vi "avgvi.vi"(11 "image in":sgl[][](array[numeric])) -> (3 "image out":sgl[][](array[numeric]))   [LabVIEW 2017]
doc: "SciScan 1.2 160622"
uses:
  GFG/GFGnumericGet.vi
  GFG/GFG library.lvlib
panel:
  in  "avg":sgl[][][](array[numeric])
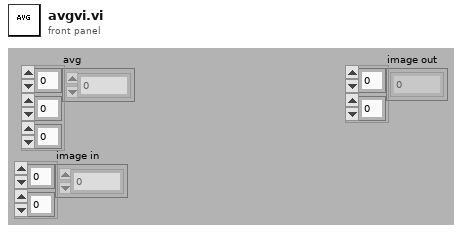
[diagram p1: front panel]
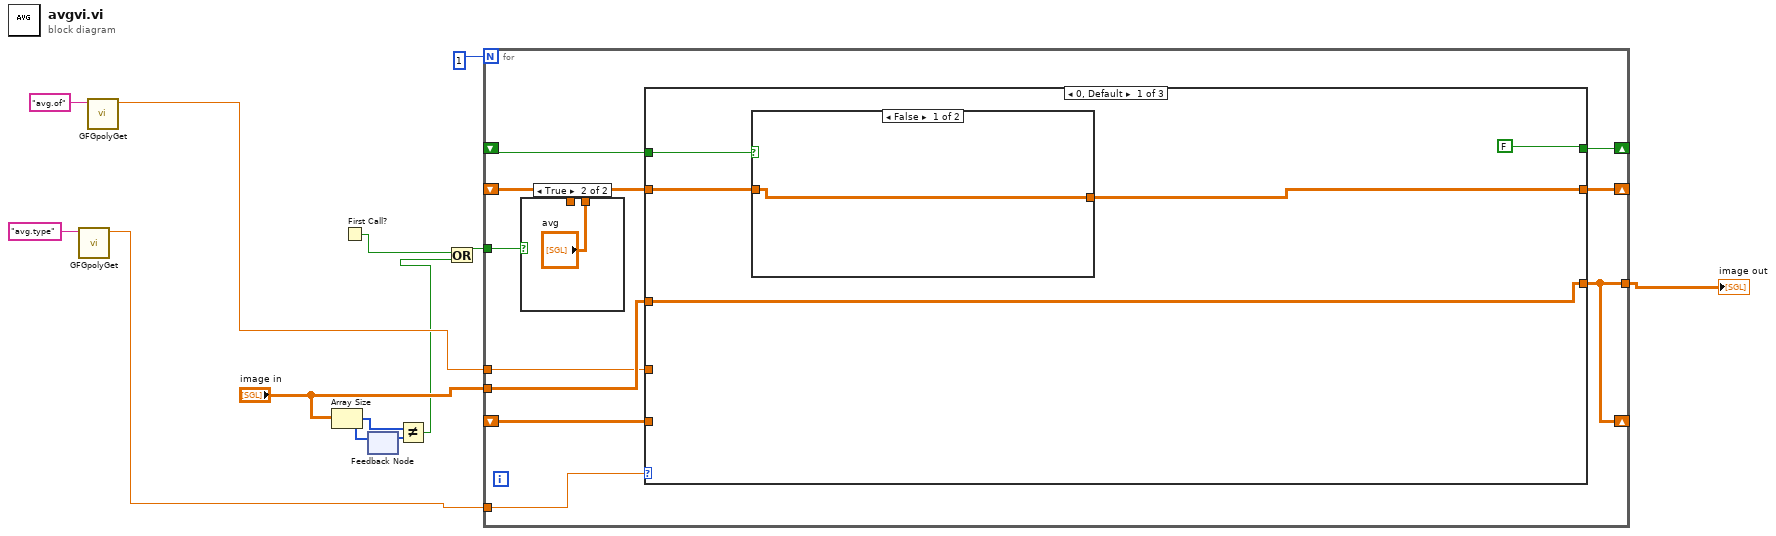
[diagram p0: block diagram]
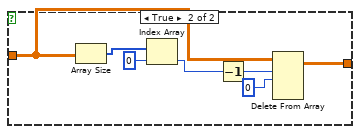
[diagram p2: hidden frame]
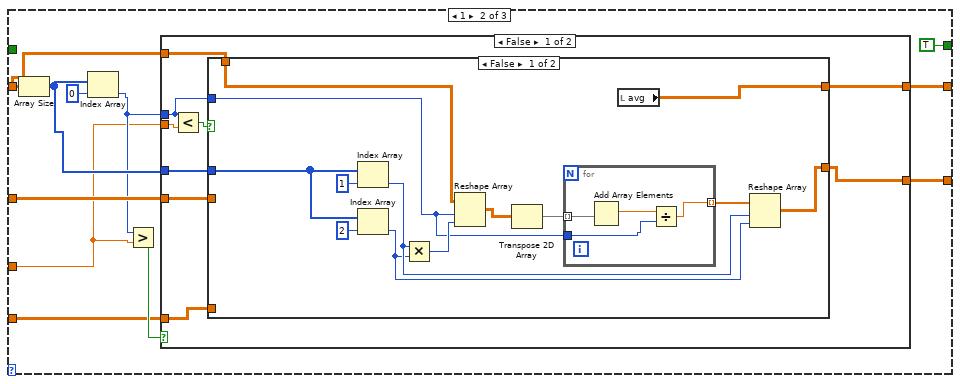
[diagram p3: hidden frame]
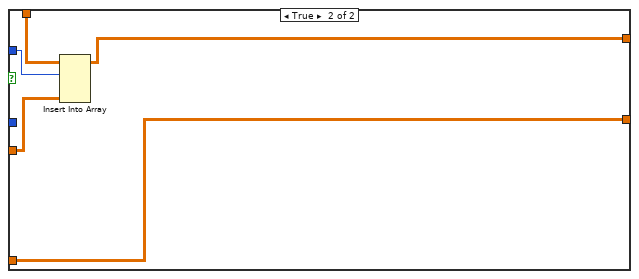
[diagram p4: hidden frame]
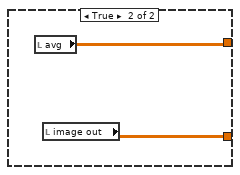
[diagram p5: hidden frame]
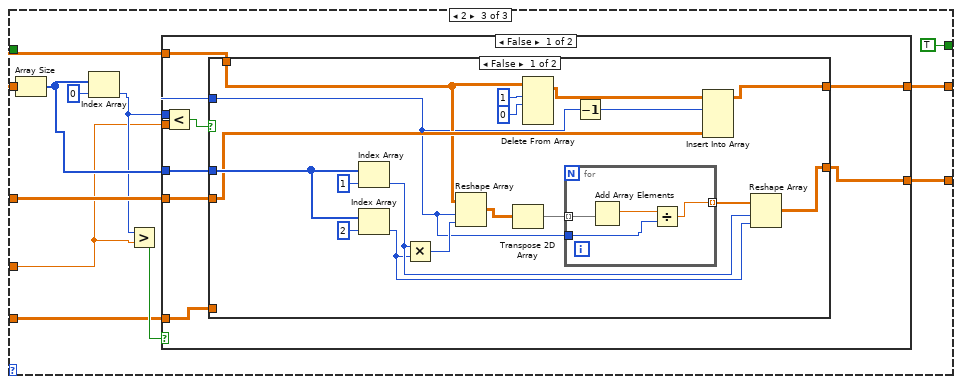
[diagram p6: hidden frame]
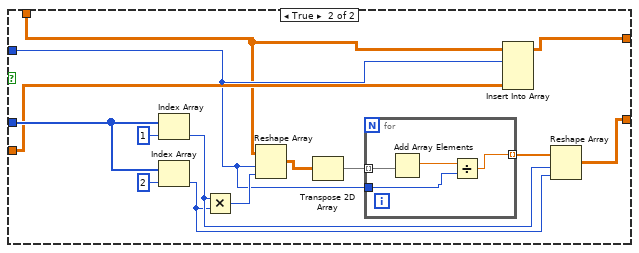
[diagram p7: hidden frame]
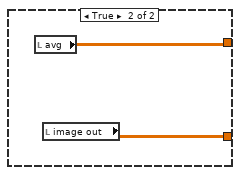
[diagram p8: hidden frame]
diagram:
  n1 = call-poly "GFGpolyGet.vi"("Variable Name in"="avg.type") -> ("Numeric"=w7:dbl)  [unwired: 8 in, 2 out]
  n2 = call-poly "GFGpolyGet.vi"("Variable Name in"="avg.of") -> ("Numeric"=w8:dbl)  [unwired: 8 in, 2 out]
  n3 = Array Size(array="image in") -> (size(s)=w6:i32[])
  n4 = First Call?() -> (First Call?: T/F=w3:bool)
  n5 = feedback #1() -> (w5:i32[])  [unwired: 1 in]
  n6 = feedback-in #1(w6) -> ()
  n7 = Not Equal?(x=w6, y=w5) -> (x != y?=w1:bool)
  n8 = Or(x=w3, y=w1) -> (x .or. y?=w2:bool)
  n9 = for {
    N: 1 -> [_]
    tunnel: "image in" -> [w23]
    shift-right: [w22] -> _
    shift-left: _ -> [w20]
    tunnel: [w17] -> w11
    tunnel: w7 -> [w19]
    tunnel: w8 -> [w18]
    shift-right: [w17] -> _
    shift-left: _ -> [w16]
    shift-right: [w14] -> _
    shift-left: _ -> [w15]
    tunnel: w2 -> [w13]
    n10 = case shown="True" w13 {
      tunnel: [w143 "avg"] -> w21
      tunnel: w20 -> [w143 _]
      frame False {
      }
      frame True {
      }
    }
    n11 = case shown="0, Default" w19 {
      tunnel: w23 -> [w28 w46 w90]
      tunnel: [w26 w45 w89] -> w22
      tunnel: w21 -> [w27 w43 w87]
      tunnel: [w28 w42 w86] -> w17
      tunnel: w18 -> [_ w39 w83]
      tunnel: w16 -> [_ w38 w82]
      tunnel: w15 -> [w25 _ _]
      tunnel: [FALSE TRUE TRUE] -> w14
      frame 0, Default {
        n12 = case shown="False" w25 {
          tunnel: w27 -> [w29 w36]
          tunnel: [w29 w35] -> w26
          frame False {
          }
          frame True {
            n13 = Array Size(array=w36) -> (size(s)=w33:i32[])
            n14 = Index Array(array=w33, index=0) -> (element=w32:i32)
            n15 = Decrement(x=w32) -> (x-1=w31:i32)
            n16 = Delete From Array(array=w36, length=w31, index (dim 0)=0 ("index (page)")) -> (array with subset deleted=w35:sgl[][][])  [unwired: 2 in, 1 out]
          }
        }
      }
      frame 1 {
        n17 = Array Size(array=w43) -> (size(s)=w44:i32[])
        n18 = Index Array(array=w44, index=0) -> (element=w41:i32)
        n19 = Greater?(x=w41, y=w39) -> (0:w40:bool)
        n20 = case shown="False" w40 {
          tunnel: w39 -> [w56 _]
          tunnel: w46 -> [w55 _]
          tunnel: w41 -> [w54 _]
          tunnel: [w53 w79] -> w45
          tunnel: w44 -> [w51 _]
          tunnel: w43 -> [w50 _]
          tunnel: [w49 w80] -> w42
          tunnel: w38 -> [w48 _]
          frame False {
            n21 = Less?(x=w54, y=w56) -> (x < y?=w52:bool)
            n22 = case shown="False" w52 {
              tunnel: w55 -> [_ w76]
              tunnel: w54 -> [w58 w78]
              tunnel: [w57 w75] -> w53
              tunnel: w50 -> [w59 w77]
              tunnel: [w60 w74] -> w49
              tunnel: w51 -> [w68 _]
              tunnel: w48 -> [_ w74]
              frame False {
                n23 = Index Array(array=w68, index=1) -> (element=w62:i32)
                n24 = Index Array(array=w68, index=2) -> (element=w61:i32)
                n25 = Multiply(x=w62, y=w61) -> (x*y=w66:i32)
                n26 = Reshape Array(w59, w58, w66) -> (w65:sgl[][])
                n27 = Transpose 2D Array(2D array=w65) -> (transposed array=w64:sgl[][])
                n28 = for {
                  tunnel: w64 -> [w73] mode=indexing
                  tunnel: w58 -> [w72]
                  tunnel: [w70] -> w63 mode=indexing
                  n29 = Add Array Elements(numeric array=w73) -> (sum=w71:sgl)
                  n30 = Divide(x=w71, y=w72) -> (x/y=w70:sgl)
                }
                n31 = local read "avg"() -> (w57:sgl[][][])
                n32 = Reshape Array(w63, w62, w61) -> (w60:sgl[][])
              }
              frame True {
                n33 = Insert Into Array(array=w77, index (dim 0)=w78, new element=w76) -> (w75:sgl[][][])  [unwired: 2 in]
              }
            }
          }
          frame True {
            n34 = local read "avg"() -> (w79:sgl[][][])
            n35 = local read "image out"() -> (w80:sgl[][])
          }
        }
      }
      frame 2 {
        n36 = Array Size(array=w87) -> (size(s)=w88:i32[])
        n37 = Index Array(array=w88, index=0) -> (element=w85:i32)
        n38 = Greater?(x=w85, y=w83) -> (0:w84:bool)
        n39 = case shown="False" w84 {
          tunnel: w83 -> [w100 _]
          tunnel: w90 -> [w99 _]
          tunnel: w85 -> [w98 _]
          tunnel: [w97 w141] -> w89
          tunnel: w88 -> [w95 _]
          tunnel: w87 -> [w94 _]
          tunnel: [w93 w142] -> w86
          tunnel: w82 -> [w92 _]
          frame False {
            n40 = Less?(x=w98, y=w100) -> (x < y?=w96:bool)
            n41 = case shown="False" w96 {
              tunnel: w99 -> [w108 w126]
              tunnel: w98 -> [w103 w124]
              tunnel: [w101 w125] -> w97
              tunnel: w94 -> [w107 w123]
              tunnel: [w109 w127] -> w93
              tunnel: w95 -> [w117 w135]
              tunnel: w92 -> [_ _]
              frame False {
                n42 = Index Array(array=w117, index=1) -> (element=w111:i32)
                n43 = Index Array(array=w117, index=2) -> (element=w110:i32)
                n44 = Multiply(x=w111, y=w110) -> (x*y=w115:i32)
                n45 = Reshape Array(w107, w103, w115) -> (w114:sgl[][])
                n46 = Transpose 2D Array(2D array=w114) -> (transposed array=w113:sgl[][])
                n47 = Delete From Array(array=w107, length=1, index (dim 0)=0 ("index (page)")) -> (array with subset deleted=w106:sgl[][][])  [unwired: 2 in, 1 out]
                n48 = for {
                  tunnel: w113 -> [w122] mode=indexing
                  tunnel: w103 -> [w121]
                  tunnel: [w119] -> w112 mode=indexing
                  n49 = Add Array Elements(numeric array=w122) -> (sum=w120:sgl)
                  n50 = Divide(x=w120, y=w121) -> (x/y=w119:sgl)
                }
                n51 = Decrement(x=w103) -> (x-1=w102:i32)
                n52 = Insert Into Array(array=w106, index (dim 0)=w102, new element=w108) -> (w101:sgl[][][])  [unwired: 2 in]
                n53 = Reshape Array(w112, w111, w110) -> (w109:sgl[][])
              }
              frame True {
                n54 = Index Array(array=w135, index=1) -> (element=w129:i32)
                n55 = Index Array(array=w135, index=2) -> (element=w128:i32)
                n56 = Multiply(x=w129, y=w128) -> (x*y=w133:i32)
                n57 = Reshape Array(w123, w124, w133) -> (w132:sgl[][])
                n58 = Transpose 2D Array(2D array=w132) -> (transposed array=w131:sgl[][])
                n59 = for {
                  tunnel: w131 -> [w140] mode=indexing
                  tunnel: w124 -> [w139]
                  tunnel: [w137] -> w130 mode=indexing
                  n60 = Add Array Elements(numeric array=w140) -> (sum=w138:sgl)
                  n61 = Divide(x=w138, y=w139) -> (x/y=w137:sgl)
                }
                n62 = Insert Into Array(array=w123, index (dim 0)=w124, new element=w126) -> (w125:sgl[][][])  [unwired: 2 in]
                n63 = Reshape Array(w130, w129, w128) -> (w127:sgl[][])
              }
            }
          }
          frame True {
            n64 = local read "avg"() -> (w141:sgl[][][])
            n65 = local read "image out"() -> (w142:sgl[][])
          }
        }
      }
    }
  }
  "image out" <- w11
